vi "LCR_Readout.vi"(8 "error in (no error)":errorcluster, 10 "Frequency in Hz":i32, 11 "WK6425 in":refnum<class "WK6425.lvclass">) -> (0 "error out":errorcluster, 1 "Resistance in Ohm":dbl format="%#_8g", 2 "Capacitance in pF":dbl, 3 "WK6425 out":refnum<class "WK6425.lvclass">)   [LabVIEW 2019, in "WK6425.lvclass"]
uses:
  WK6425.lvclass
  C:/Users/probe/Desktop/TRIUMF-Dark-Box/InstrControl/InstrControl.lvclass
  InstrControl.lvclass
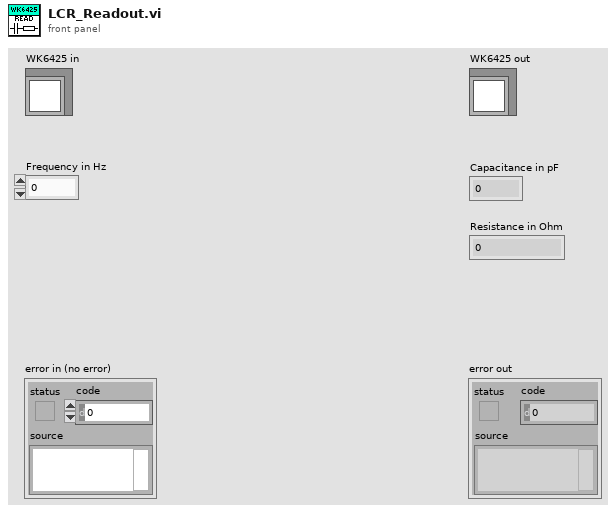
[diagram p1: front panel]
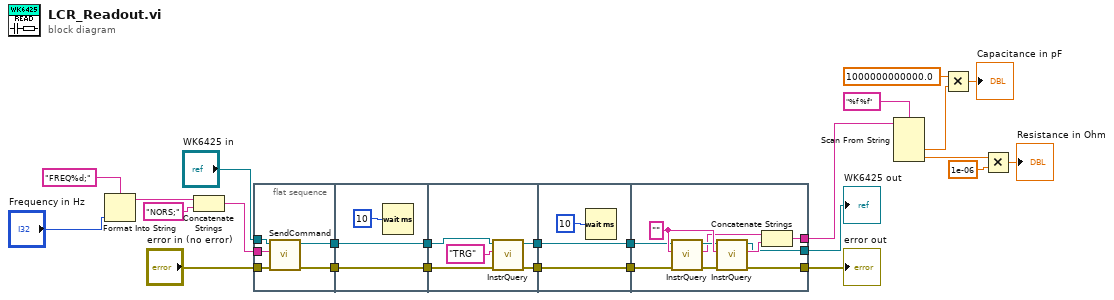
[diagram p0: block diagram]
diagram:
  n1 = Format Into String(format string="FREQ%d;", "Frequency in Hz") -> (resulting string=w19:string)  [unwired: 2 in, 1 out]
  n2 = Concatenate Strings(w19, "NORS;") -> (w20:string)
  n3 = flat-sequence {
    tunnel: w20 -> [w28]
    tunnel: "error in (no error)" -> [w30]
    tunnel: "WK6425 in" -> [w26]
    tunnel: [w29] -> w24
    tunnel: [w27] -> w23
    tunnel: w24 -> [w32]
    tunnel: [w32] -> w22
    tunnel: w23 -> [w31]
    tunnel: [w31] -> w21
    tunnel: w22 -> [w38]
    tunnel: w21 -> [w36]
    tunnel: [w35] -> w3
    tunnel: [w34] -> w1
    tunnel: [w40] -> w4
    tunnel: w3 -> [w40]
    tunnel: [w39] -> w2
    tunnel: w1 -> [w39]
    tunnel: [w42] -> w10
    tunnel: [w43] -> w13
    tunnel: [w44] -> w9
    tunnel: w4 -> [w46]
    tunnel: w2 -> [w45]
    frame #0 {
      n4 = call "SendCommand.vi"("error in (no error)"=w30, "Command string"=w28, "InstControl in"=w26) -> ("error out"=w29:errorcluster, "InstControl out"=w27:refnum<class "WK6425.lvclass">)  [unwired: 7 in]
    }
    frame #1 {
      n5 = Wait (ms)(milliseconds to wait=10) -> ()  [unwired: 1 out]
    }
    frame #2 {
      n6 = call-dynamic "InstrQuery.vi"("error in (no error)"=w38, "Command string"="TRG", "InstControl in"=w36) -> ("error out"=w34:errorcluster, "InstControl out"=w35:refnum<class "WK6425.lvclass">)  [unwired: 6 in, 1 out]
    }
    frame #3 {
      n7 = Wait (ms)(milliseconds to wait=10) -> ()  [unwired: 1 out]
    }
    frame #4 {
      w51 = ""
      n8 = call-dynamic "InstrQuery.vi"("error in (no error)"=w45, "Command string"=w51, "InstControl in"=w46) -> ("error out"=w50:errorcluster, "Instrument response"=w48:string, "InstControl out"=w49:refnum<class "WK6425.lvclass">)  [unwired: 6 in]
      n9 = call-dynamic "InstrQuery.vi"("error in (no error)"=w50, "Command string"=w51, "InstControl in"=w49) -> ("error out"=w44:errorcluster, "Instrument response"=w47:string, "InstControl out"=w42:refnum<class "WK6425.lvclass">)  [unwired: 6 in]
      n10 = Concatenate Strings(w48, w47) -> (w43:string)
    }
  }
  n11 = Scan From String(format string="%f %f", input string=w13) -> (output 1=w14:dbl, output 2=w6:dbl)  [unwired: 4 in, 3 out]
  n12 = Multiply(x=1000000000000.0 ("y"), y=w14) -> (x*y=→"Capacitance in pF":dbl)
  n13 = Multiply(x=w6, y=1e-06) -> (x*y=→"Resistance in Ohm":dbl)
  "error out" <- w9
  "WK6425 out" <- w10
